vi "Untitled 1.vi"() -> ()   [LabVIEW 2022 SP3, in "ADS_Library.lvlib"]
uses:
  ADS_Library.lvlib
  <userlib>/Beckhoff-LabVIEW-Interface/Utilities/Notification/Buffered User-Event Data.ctl
  <userlib>/Beckhoff-LabVIEW-Interface/_DependsOn/Base/Read/Register E-Notification Buffered.vi
panel:
  out "Waveform Chart":sgl(graph)
  out "SymbolName":string
  out "Has started?":bool
  in  "Stop Notifications":bool
  out "Has stopped?":bool
  in  "Start Notifications":bool=TRUE
  out "error out":errorcluster
  in  "error in":errorcluster
  in  "String":string="<PortInfo><Inputs><SymbolControlItems /></Inputs><Outputs><SymbolControlItems><SymbolControlItem GroupName=\"ADS Read\" GroupDescription=\"Parameters for ADS Read command\"><Parameters><Parameter Name=\"Name\">Term 9 (ELM3704-0000).PAI SamplesR32 1 Channel 1.Samples</Parameter><Parameter Name=\"SymbolName\">Term 9 (ELM3704-0000).PAI SamplesR32 1 Channel 1.Samples</Parameter><Parameter Name=\"SymbolType\">Samples_9BD8E00D</Parameter><Parameter Name=\"SymbolGuid\"></Parameter><Parameter Name=\"AmsNetId\">192.168.80.50.1.1</Parameter><Parameter Name=\"Port\">27906</Parameter><Parameter Name=\"IndexGroup\">#x0</Parameter><Parameter Name=\"IndexOffset\">#x0</Parameter><Parameter Name=\"BitSize\">32</Parameter><Parameter Name=\"CycleTime [ms]\">1</Parameter><Parameter Name=\"Transmode\">3</Parameter><Parameter Name=\"Timeout [ms]\">1000</Parameter><Parameter Name=\"TCBufferSize [Samples]\">10</Parameter><Parameter Name=\"LVBufferSize [Samples]\">50</Parameter><Parameter Name=\"Expected min delay [ms]\">50</Parameter></Parameters></SymbolControlItem></SymbolControlItems></Outputs></PortInfo>"
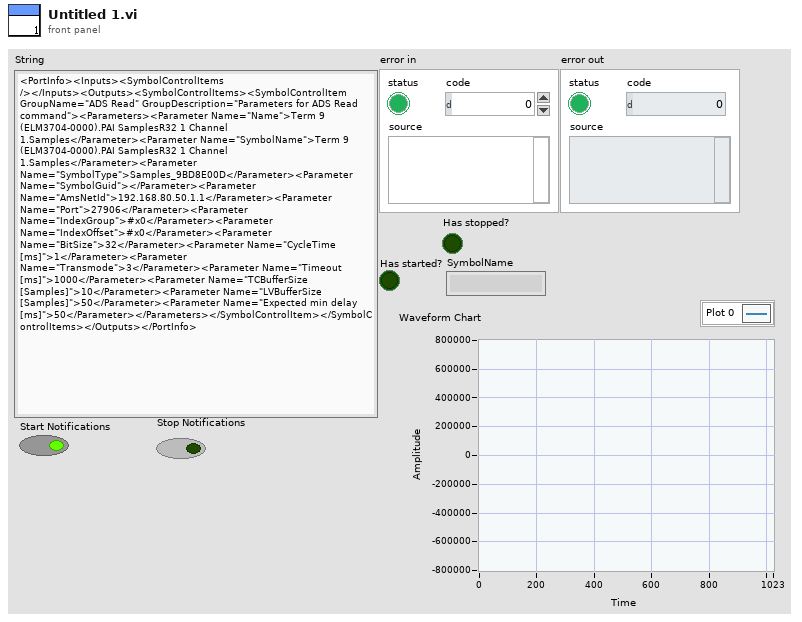
[diagram p1: front panel]
types:
  T1 = typedef "Buffered User-Event Data.ctl" = cluster{"NotiHandle":u32, "Samples":i32, "BufferInfo":cluster{"Previous Overflow Samples":u32, "Missing Samples":u32, "Buffer Usage":dbl}, "RawData":u8[], "Timestamps":i64[]}
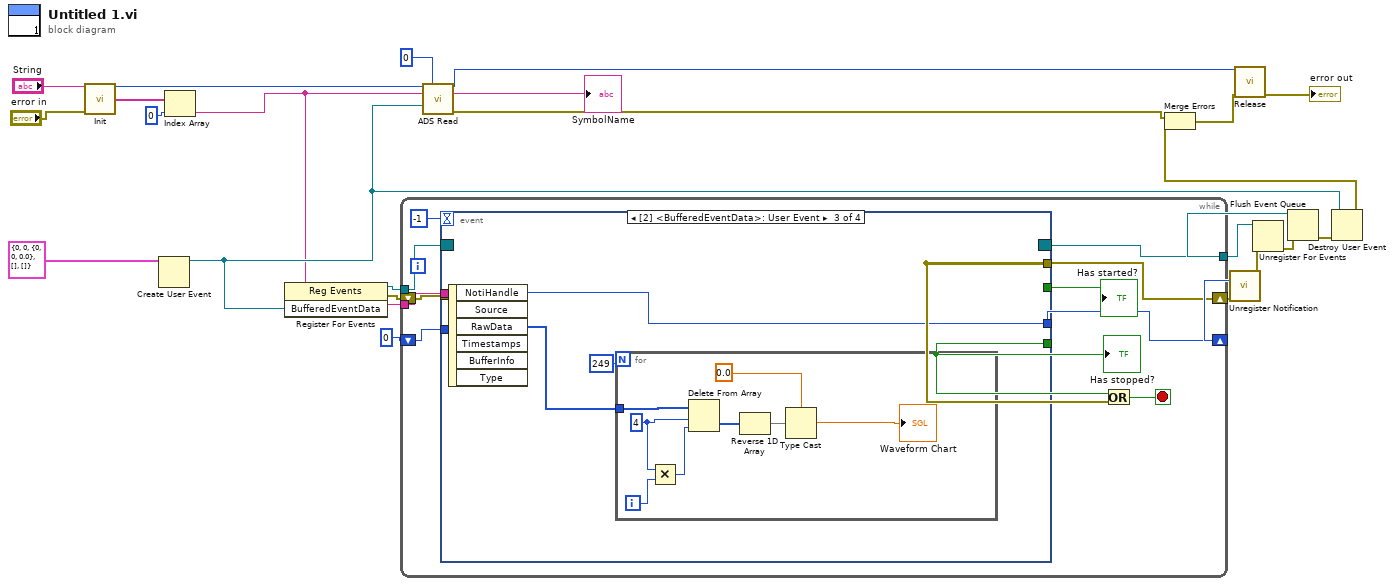
[diagram p0: block diagram]
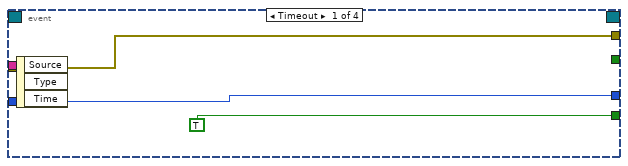
[diagram p2: hidden frame]
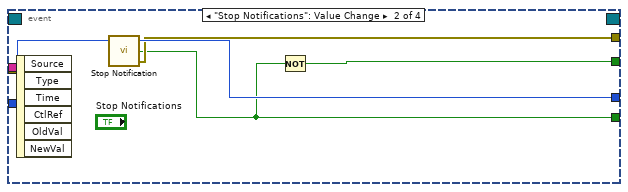
[diagram p3: hidden frame]
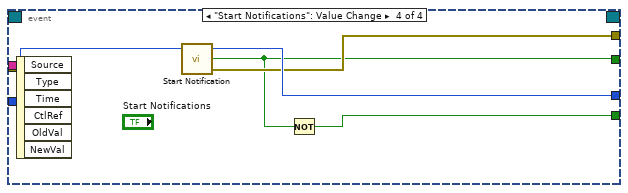
[diagram p4: hidden frame]
diagram:
  n1 = call <userlib>:"Init.vi"("XMLDescription"="String", "error in (no error)"="error in") -> ("Handle"=w3:u32, "ReadGrpSymbols"=w23:string[])  [unwired: 9 in, 3 out]
  n2 = Create User Event(user event datatype=T1 {"NotiHandle"=0, "Samples"=0, "BufferInfo"={"Previous Overflow Samples"=0, "Missing Samples"=0, "Buffer Usage"=0.0}, "RawData"=[], "Timestamps"=[]} ("BufferedEventData")) -> (user event=w12:refnum<user-event>)  [unwired: 1 in, 1 out]
  n3 = Index Array(array=w23, index=0) -> (element=w4:string)
  n4 = register-events(w12) -> (reference out=w17:refnum<event-registration>, error out=w7:errorcluster)  [unwired: 2 in]
  n5 = while {
    tunnel: w17 -> [w34]
    shift-right: [w32] -> w5
    shift-left: u32 0 ("NotiHandle") -> [w33]
    tunnel: [w31] -> w13
    shift-right: [w29] -> w6
    shift-left: w7 -> [w30]
    tunnel: w4 -> [w27]
    stop <- w28 stop-if-true
    n6 = event shown="[2] <BufferedEventData>: User Event" {
      selector: w34 -> [_ _ _ _]
      dyn-events: [_ _ _ _] -> w31
      timeout: -1 -> [_ _ _ _]
      tunnel: w33 -> [w38 w43 _ w58]
      tunnel: [w38 w42 w46 w59] -> w32
      tunnel: [TRUE ("Has stopped?") w39 _ w56] -> w25
      tunnel: w30 -> [w37 _ _ _]
      tunnel: [w37 w41 _ w57] -> w29
      tunnel: w27 -> [_ _ _ _]
      tunnel: [_ w40 _ w55] -> w26
      event Timeout {
        n7 = event-data() -> ()  [unwired: 1 in, 3 out]
      }
      event "Stop Notifications": Value Change {
        n8 = event-data() -> ()  [unwired: 1 in, 6 out]
        n9 = call <userlib>:"Stop Notification.vi"("Reader Handle"=w43) -> ("error out"=w41:errorcluster, "Has stopped?"=w39:bool, "Reader Handle"=w42:u32)  [unwired: 2 in]
        n10 = Not(x=w39) -> (.not. x?=w40:bool)
      }
      event User Event {
        n11 = event-data() -> ("NotiHandle"=w46:u32, "RawData"=w44:u8[])  [unwired: 1 in, 4 out]
        n12 = for {
          N: 249 -> [_]
          tunnel: w44 -> [w54]
          i -> [w53]
          w52 = 4 ("length")
          n13 = Multiply(x=w52, y=w53) -> (x*y=w51:i32)
          n14 = Delete From Array(array=w54, length=w52, index=w51) -> (deleted portion=w49:u8[])  [unwired: 1 out]
          n15 = Reverse 1D Array(array=w49) -> (reversed array=w50:u8[])
          n16 = Type Cast(type=sgl 0.0, x=w50) -> (*(type *) &x=→"Waveform Chart":sgl)
        }
      }
      event "Start Notifications": Value Change {
        n17 = event-data() -> ()  [unwired: 1 in, 6 out]
        n18 = call <userlib>:"Start Notification.vi"("Reader Handle"=w58) -> ("error out"=w57:errorcluster, "Has started?"=w55:bool, "Reader Handle"=w59:u32)  [unwired: 2 in]
        n19 = Not(x=w55) -> (.not. x?=w56:bool)
      }
    }
    "Has stopped?" <- w25
    "Has started?" <- w26
    n20 = Or(x=w25, y=w29) -> (x .or. y?=w28:bool)
  }
  n21 = call-poly <userlib>:"ADS Read.vi"("Handle"=w3, "ElapseTimeMs"=u64 0, "SymbolName"=w4, "Noti. E-Buffered Event Ref"=w12) -> ("Handle"=w9:u32, "SymbolName"=→"SymbolName":string, "error out"=w11:errorcluster)  [unwired: 9 in]
  n22 = call <userlib>:"Unregister Notification.vi"("Reader Handle"=w5, "error in"=w6) -> ("error out"=w8:errorcluster)  [unwired: 10 in, 3 out]
  n23 = Flush Event Queue(0:w13, 3:w8) -> (11:w14:errorcluster)  [unwired: 4 in, 2 out]
  n24 = Unregister For Events(event registration refnum=w13, error in=w14) -> (error out=w15:errorcluster)
  n25 = Destroy User Event(user event=w12, error in=w15) -> (error out=w10:errorcluster)
  n26 = Merge Errors(w11, w10) -> (w19:errorcluster)
  n27 = call <userlib>:"Release.vi"("Handle"=w9, "error in (no error)"=w19) -> ("error out"=→"error out":errorcluster)  [unwired: 13 in]
